vi "DVB Demonstrator.vi"() -> ()   [LabVIEW 2011]
panel:
  in  "Threshold":dbl=0.5
  in  "Joystick Input":dbl(slide)=0.005128205128205127 scale=-1.0..1.0
  out "Value":dbl
  in  "Bump Quanta":dbl=5.0
  in  "Initial Count":i64
  in  "Reset":bool
  out "Count":i64
  in  "stop":bool
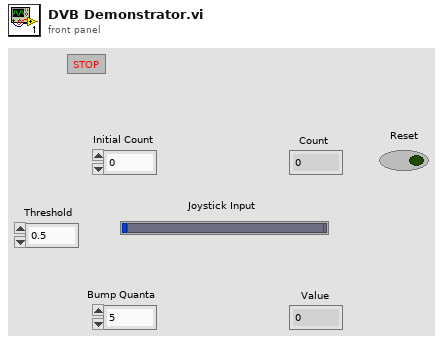
[diagram p1: front panel]
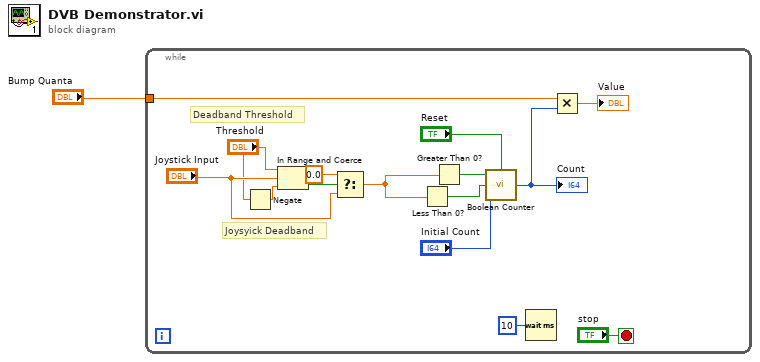
[diagram p0: block diagram]
diagram:
  n1 = while {
    tunnel: "Bump Quanta" -> [w12]
    stop <- "stop" stop-if-true
    # "Deadband Threshold"
    # "Joysyick Deadband"
    n2 = Negate(x="Threshold") -> (-x=w9:dbl)
    n3 = In Range and Coerce(upper limit="Threshold", x="Joystick Input", lower limit=w9) -> (In Range?=w8:bool)  [unwired: 1 out]
    n4 = Select(t=0.0, s=w8, f="Joystick Input") -> (s? t:f=w3:dbl)
    n5 = Less Than 0?(x=w3) -> (x < 0?=w4:bool)
    n6 = Greater Than 0?(x=w3) -> (x > 0?=w5:bool)
    n7 = call "Boolean Counter.vi"("Reset"="Reset", "Initial Count"="Initial Count", "Down"=w4, "Up"=w5) -> ("Count"=w11:i64)
    "Count" <- w11
    n8 = Wait (ms)(milliseconds to wait=u32 10) -> ()  [unwired: 1 out]
    n9 = Multiply(x=w12, y=w11) -> (x*y=→"Value":dbl)
  }
